vi "Get Variant.vi"(8 "error in (no error)":errorcluster, 11 "VariantMessage In":refnum<class "VariantMessage.lvclass">) -> (0 "error out":errorcluster, 2 "Message Data":variant, 3 "VariantMessage Out":refnum<class "VariantMessage.lvclass">)   [LabVIEW 2009, in "LapDog.Messaging.v2.NativeTypes.lvlib" / "VariantMessage.lvclass"]
doc: "Returns the data contained in the message.\n\nThis method executes regardless of the error in state."
uses:
  VariantMessage.lvclass
  VariantMessage.lvclass/VariantMessage.ctl
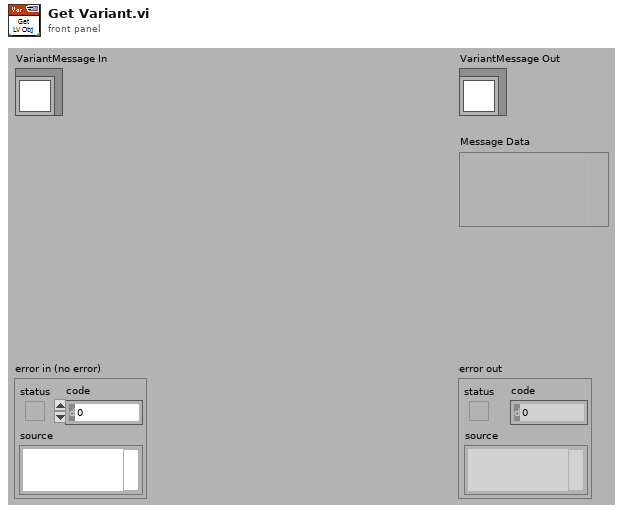
[diagram p1: front panel]
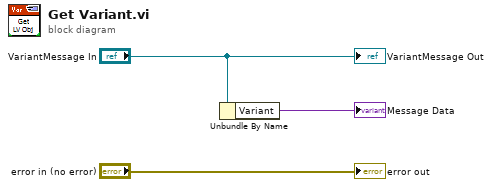
[diagram p0: block diagram]
diagram:
  n1 = Unbundle By Name("VariantMessage In") -> ("Variant"=→"Message Data":variant)
  "error out" <- "error in (no error)"
  "VariantMessage Out" <- "VariantMessage In"
